vi "motor.vi"() -> ()   [LabVIEW 2017]
panel:
  in  "stop":bool
  in  "Stop Button":bool
  in  "Duty Cycle (-100 to + 100)":dbl
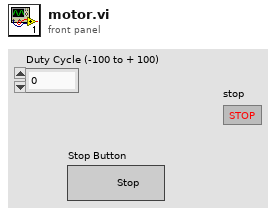
[diagram p1: front panel]
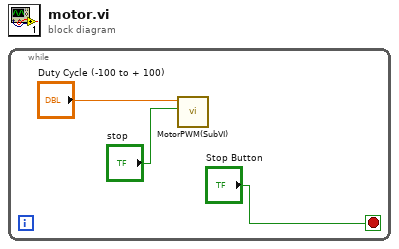
[diagram p0: block diagram]
diagram:
  n1 = while {
    stop <- "Stop Button" stop-if-true
    n2 = call "MotorPWM(SubVI).vi"("Stop Vi"="stop", "Duty Cycle (-100 to + 100)"="Duty Cycle (-100 to + 100)") -> ()  [unwired: 10 in]
  }
